vi "Execute.vi"(8 "error in (no error)":errorcluster, 11 "LP Filter in":refnum<class "LP Filter.lvclass">) -> (0 "error out":errorcluster, 2 "Data":dbl[](array[numeric]), 3 "LP Filter out":refnum<class "LP Filter.lvclass">)   [LabVIEW 2021, in "LP Filter.lvclass"]
uses:
  LP Filter.lvclass
  <vilib>/Analysis/3filter.llb/Butterworth Filter (DBL).vi
  Decorator/Decorator.lvclass
  LP Filter.lvclass/LP Filter.ctl
  <vilib>/Analysis/NI_AALBase.lvlib
  C:/PPLs/Decorator-Pattern/decorator-main/Presentation/Decorator/Decorator.lvclass
  C:/PPLs/Decorator-Pattern/decorator-main/Presentation/Component/Component.lvclass
  C:/PPLs/Decorator-Pattern/decorator-main/Presentation/LP Filter/LP Filter.lvclass
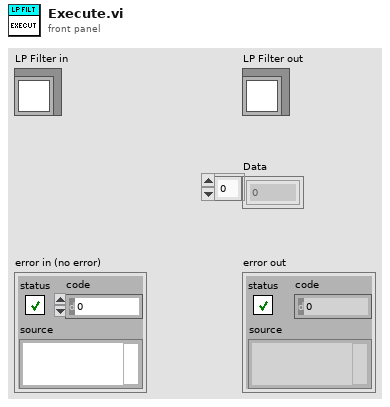
[diagram p1: front panel]
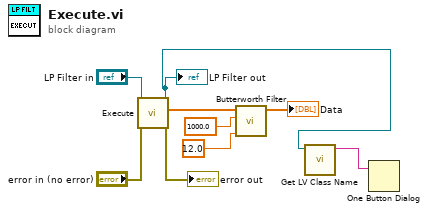
[diagram p0: block diagram]
diagram:
  n1 = call-parent "Execute.vi"("error in (no error)"="error in (no error)", "Decorator in"="LP Filter in") -> ("error out"=→"error out":errorcluster, "Data"=w6:dbl[], "Decorator out"=w1:refnum<class "LP Filter.lvclass">)  [unwired: 7 in]
  "LP Filter out" <- w1
  n2 = call-poly <vilib>:"Butterworth Filter.vi"("low cutoff freq: fl"=12.0, "sampling freq: fs"=1000.0, "X"=w6) -> ("Filtered X"=→"Data":dbl[])  [unwired: 5 in, 1 out]
  n3 = call <vilib>:"Get LV Class Name.vi"("object"=w1) -> ("class name"=w2:string)  [unwired: 9 in, 1 out]
  n4 = One Button Dialog(message=w2) -> ()  [unwired: 1 in, 1 out]
